vi "MoveLiftIncre.vi"(8 "error in (no error)":errorcluster, 10 "Distance (in)":dbl) -> (0 "error out":errorcluster)   [LabVIEW 2015]
uses:
  TW Global.vi
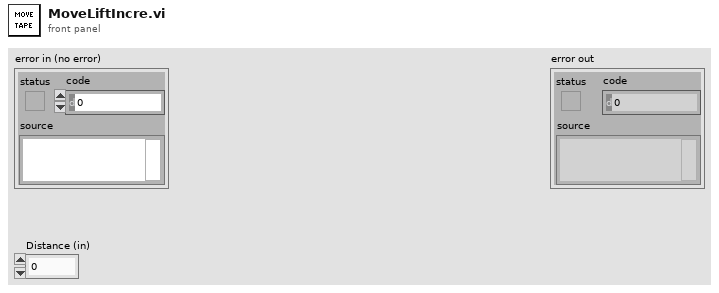
[diagram p1: front panel]
types:
  T1 = typedef "Detailed Motor Type Def.ctl" = cluster{"MotorRef":T2, "Encoder Ticks Per Rev":dbl, "Set Position":dbl, "Wheel Radius":dbl}
  T2 = typedef "WPI_MotorControlDeviceRef.ctl" = cluster{"DeviceStatus":errorcluster, "Type":T3, "PWM":cluster{"PWM Channel":T4, "DeadBand":T5}, "CAN":cluster{"Device Number":u8, "Control Mode":T6, "Semaphore":T7, "Max Vout":dbl, "TalonSRX Control Mode":T8}, "Invert":bool}
  T3 = typedef "WPI_MotorControlType.ctl" = enum16{"PWM", "CAN", "CANTalonSRX"}
  T4 = typedef "FPGA_DIOPWMChannel.ctl" = enum8{"PWM 0", "PWM 1", "PWM 2", "PWM 3", "PWM 4", "PWM 5", "PWM 6", "PWM 7", "PWM 8", "PWM 9", "PWM MXP 0", "PWM MXP 1", "PWM MXP 2", "PWM MXP 3", "PWM MXP 4", "PWM MXP 5", "PWM MXP 6", "PWM MXP 7", "PWM MXP 8", "PWM MXP 9", "Invalid"}
  T5 = typedef "WPI_PWMDeadband.ctl" = cluster{"Name":string, "maxPositivePwm":i32, "minPositivePwm":i32, "centerPwm":i32, "maxNegativePwm":i32, "minNegativePwm":i32, "angularRange":u16}
  T6 = typedef "WPI_CANJaguar_ControlMode.ctl" = enum8{"Percent VBus", "Current", "Speed", "Position", "Voltage"}
  T7 = typedef "Semaphore RefNum" = refnum<k1>
  T8 = typedef "WPI_CANTalonSRX_APIControlMode.ctl" = enum8{"Percent VBus", "Speed", "Position", "Slave", "Unchanged / Invalid", "Voltage Compensation", "Current", "Motion Profile"}
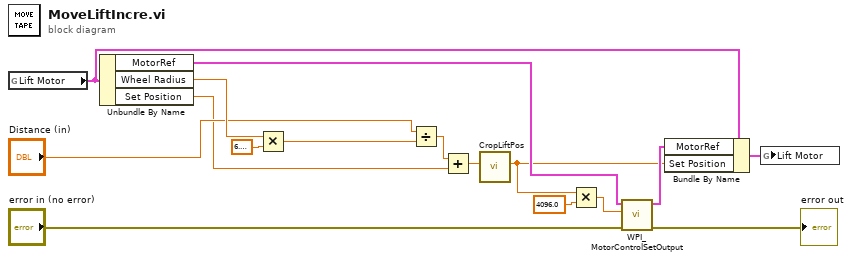
[diagram p0: block diagram]
diagram:
  n1 = global read "TW Global.vi" "Lift Motor"() -> (w5:T1)
  n2 = Unbundle By Name(w5) -> ("MotorRef"=w8:T2, "Wheel Radius"=w15:dbl, "Set Position"=w11:dbl)
  n3 = Multiply(x=w15, y=6.283185307179586) -> (x*y=w14:dbl)
  n4 = Divide(x="Distance (in)", y=w14) -> (x/y=w12:dbl)
  n5 = Add(x=w12, y=w11) -> (x+y=w2:dbl)
  n6 = call "CropLiftPos.vi"("Position"=w2) -> ("New Position"=w1:dbl)  [unwired: 10 in]
  n7 = Multiply(x=w1, y=4096.0) -> (x*y=w9:dbl)
  n8 = call <vilib>:"WPI_MotorControlSetOutput.vi"("error in (no error)"="error in (no error)", "Output"=w9, "MotorControlDevRef"=w8) -> ("error out"=→"error out":errorcluster, "MotorControlDevRef"=w4:T2)  [unwired: 6 in, 1 out]
  n9 = Bundle By Name(cluster=w5, "MotorRef"=w4, "Set Position"=w1) -> (w3:T1)
  n10 = global write "TW Global.vi" "Lift Motor"(w3) -> ()
